vi "LDA_An_mx.vi"(0 "Board type":T1=enum."NI-DAQmx", 1 "interval scanning":bool, 2 "Client Time":dbl=3298049951.624875, 5 "No of samples+extra":i32=1024 min=0 step=1, 7 "Trigger mode":T2, 9 "output polarity":u16(ring)=1 items=["do not change", "positive", "negative"], 11 "Ch & spans":T3[](array[typedef]) {"low limit (-10V)" format="%.3f"; "high limit (10V)" format="%.3f"}, 12 "Actual Sampling rate (Hz)":dbl=100000.0 format="%.2f", 13 "Local Client?":bool=TRUE, 14 "Current Block No":i32) -> (3 "LDA Binary output":u16[][](array[numeric]), 4 "I16 Analogue data block":i16[][](array[numeric]), 6 "I16 TOF block (mu.s)":i16[](array[numeric]), 8 "Block Timings":T4={"Started"=3298049951.656125, "Ended"=3298049951.67175, "Analogue Frequency Hz"=100000.0} {"Analogue Frequency Hz" format="%.2f"}, 10 "group channel settings":T5(array[cluster]) {"scale offset" format="%#_16f"; "scale multiplier" format="%#_16f"; "input mode" format="%#_16f"; "coupling" format="%#_16f"; "gain" format="%#_16f"; "polarity" format="%#_16f"; "range" format="%#_16f"; "lower input limits" format="%#_16f"; "upper input limits" format="%#_16f"}, 15 "error out":errorcluster)   [LabVIEW 2011]
uses:
  PWAtasksGLOBAL.vi
  <vilib>/DAQmx/configure/timing.llb/DAQmx Timing (Sample Clock).vi
  <vilib>/DAQmx/create/channels.llb/DAQmx Create Channel (AI-Voltage-Basic).vi
  Globals/Meas_global.vi
  Controls/Block_start_and_end.ctl
  Applications/National Instruments/LabVIEW 2011/resource/objmgr/daqmx.rc
  <vilib>/DAQmx/read.llb/DAQmx Read (Analog 2D DBL NChan NSamp).vi
  Globals/LDA_meas_global_2.vi
  Controls/Ch_and_Spans.ctl
  Controls/Trigger_Mode.ctl
  Controls/Board_Types.ctl
panel:
  out "AI.Voltage.Rngs":dbl[](array[numeric])=[-10.0, 10.0]
  out "TotalSampPerChanAcquired":dbl=1024.0
  out "AvailSampPerChan":u32
  out "CurrReadPos":dbl=1024.0
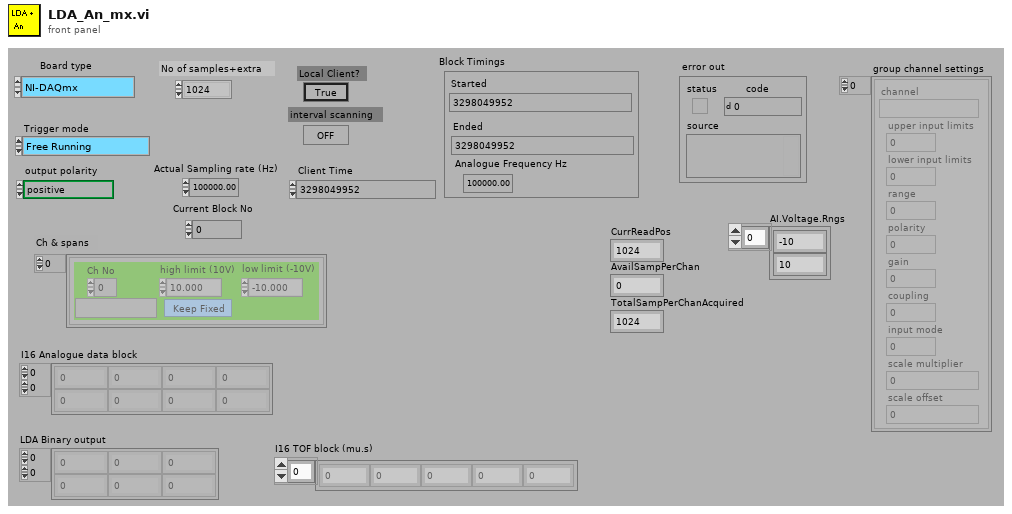
[diagram p1: front panel]
types:
  T1 = typedef "Board_Types.ctl" = enum16{"Simulate", "Local ADAM", "Server ADAM", "NI-DAQmx", "NI-DAQmxBase", "ADC488", "DT LV-link"}
  T2 = typedef "Trigger_Mode.ctl" = enum16{"Free Running", "Start on Trigger", "Trigger Every Block", "Trigger Every Sample"}
  T3 = typedef "Ch_and_Spans.ctl" = cluster{"high limit (10V)":sgl, "low limit (-10V)":sgl, "Ch No":i16, "Var name":string, "Use Latest Calib":bool}
  T4 = typedef "Block_start_and_end.ctl" = cluster{"Started":dbl, "Ended":dbl, "Analogue Frequency Hz":dbl}
  T5 = cluster{"channel":string, "upper input limits":sgl, "lower input limits":sgl, "range":sgl, "polarity":u16, "gain":sgl, "coupling":u16, "input mode":u16, "scale multiplier":dbl, "scale offset":dbl}[]
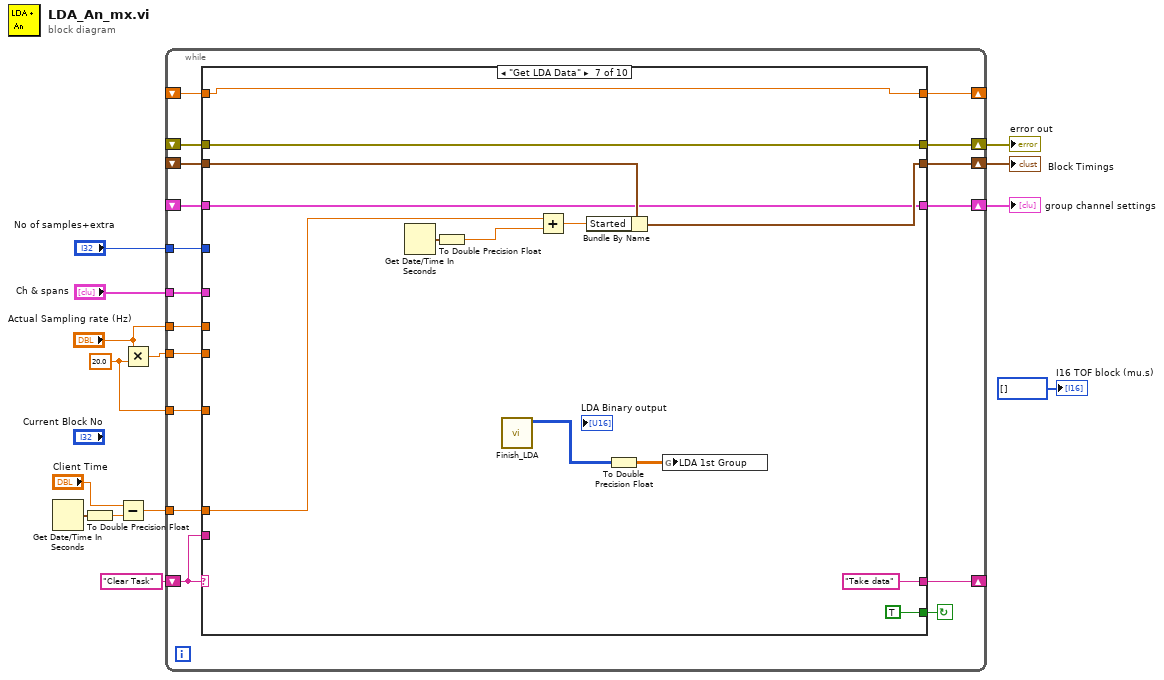
[diagram p0: block diagram]
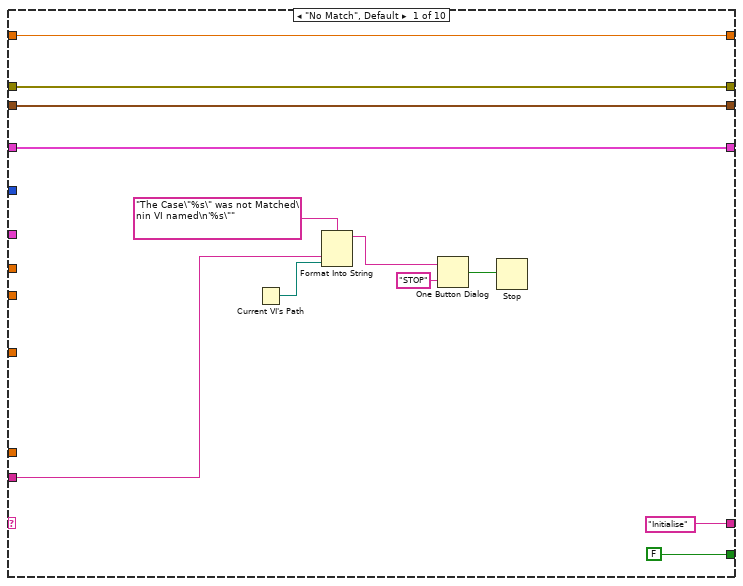
[diagram p2: hidden frame]
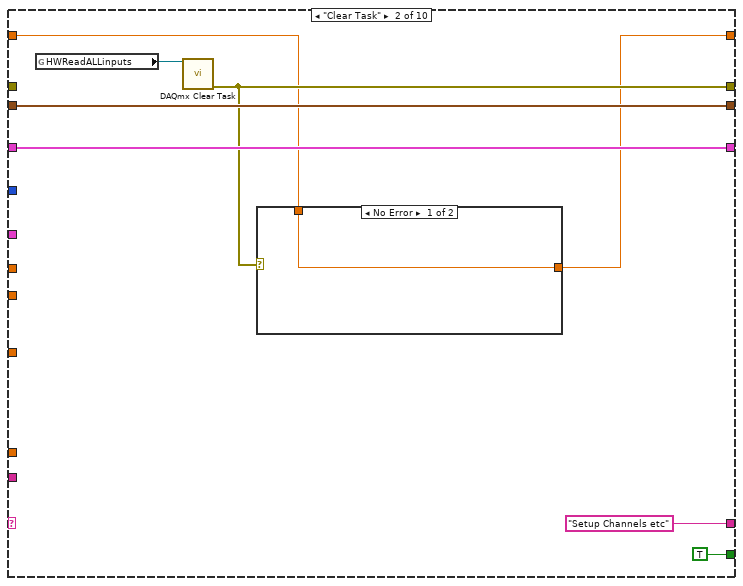
[diagram p3: hidden frame]
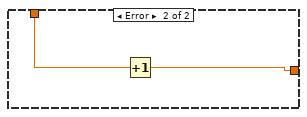
[diagram p4: hidden frame]
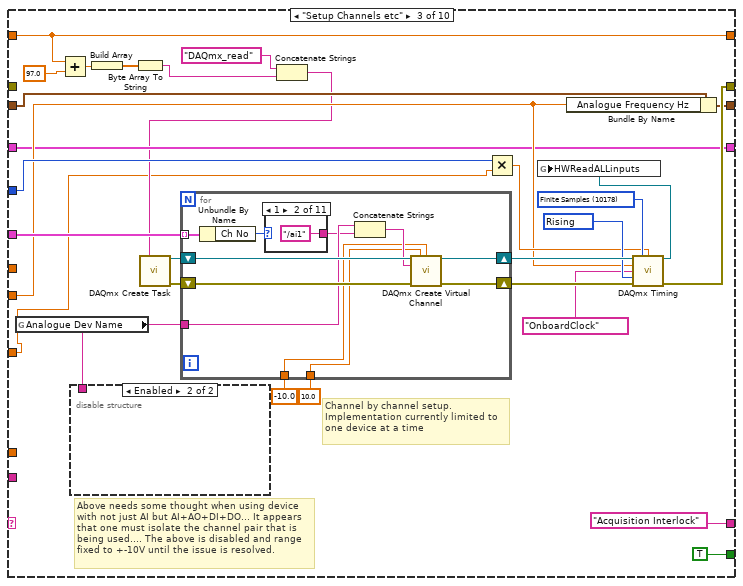
[diagram p5: hidden frame]
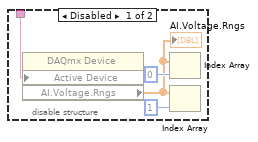
[diagram p6: hidden frame]
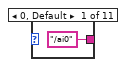
[diagram p7: hidden frame]
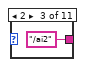
[diagram p8: hidden frame]
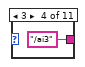
[diagram p9: hidden frame]
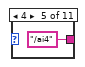
[diagram p10: hidden frame]
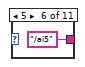
[diagram p11: hidden frame]
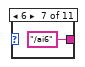
[diagram p12: hidden frame]
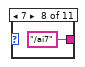
[diagram p13: hidden frame]
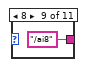
[diagram p14: hidden frame]
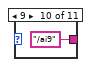
[diagram p15: hidden frame]
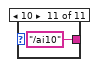
[diagram p16: hidden frame]
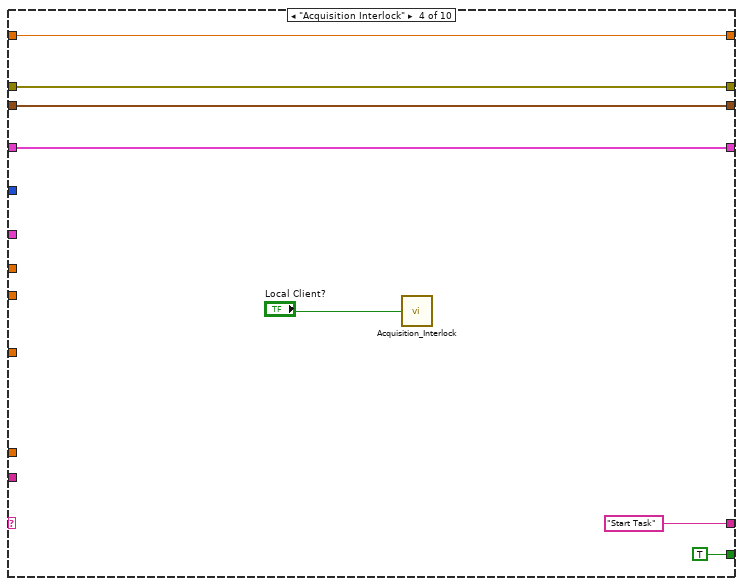
[diagram p17: hidden frame]
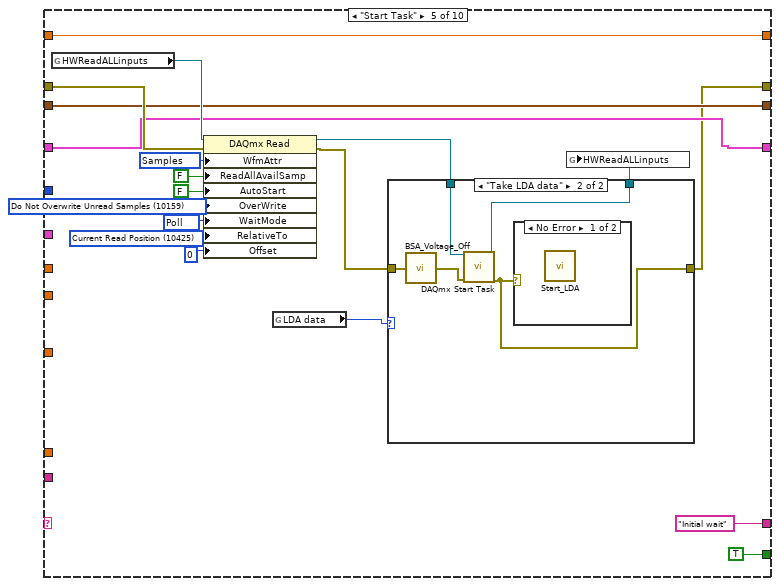
[diagram p18: hidden frame]
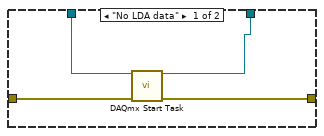
[diagram p19: hidden frame]
diagram:
  w1 = 20.0 ("y")
  n1 = Get Date/Time In Seconds() -> (seconds since 1Jan1904=w13:timestamp)
  n2 = To Double Precision Float(number=w13) -> (double precision float=w12:dbl)
  n3 = Subtract(x="Client Time", y=w12) -> (x-y=w10:dbl)
  n4 = Multiply(x="Actual Sampling rate (Hz)", y=w1) -> (x*y=w3:dbl)
  n5 = while {
    shift-left: "Clear Task" -> [w29]
    shift-right: [w30] -> _
    shift-right: [w21] -> w6
    shift-left: _ -> [w28]
    shift-right: [w20] -> w7
    shift-left: _ -> [w27]
    tunnel: w10 -> [w26]
    tunnel: w3 -> [w25]
    tunnel: "No of samples+extra" -> [w24]
    tunnel: "Ch & spans" -> [w23]
    shift-right: [w19] -> w5
    shift-left: _ -> [w22]
    shift-right: [w18] -> _
    shift-left: _ -> [w17]
    tunnel: "Actual Sampling rate (Hz)" -> [w16]
    tunnel: w1 -> [w15]
    stop <- w31 continue-if-true
    n6 = case shown="\"Get LDA Data\"" w29 {
      tunnel: [FALSE TRUE TRUE TRUE TRUE TRUE TRUE TRUE FALSE FALSE] -> w31
      tunnel: ["Initialise" "Setup Channels etc" "Acquisition Interlock" "Start Task" "Initial wait" "Get LDA Data" ("f") "Take data" "End Time" "End" ("f") "End" ("f")] -> w30
      tunnel: w29 -> [w38 _ _ _ _ _ _ _ _ _]
      tunnel: [w35 w46 w77 w114 w118 w153 w170 w190 w199 w212] -> w21
      tunnel: w28 -> [w35 _ _ w114 w126 w153 w170 w196 w199 w212]
      tunnel: [w33 w50 w75 w112 w125 w146 w174 w197 w205 T4 {"Started"=0.0, "Ended"=0.0, "Analogue Frequency Hz"=1000.0} ("Block Timings")] -> w20
      tunnel: w27 -> [w33 w50 w76 w112 w125 w147 w175 w197 w206 _]
      tunnel: w26 -> [_ _ _ _ _ w145 w172 _ w203 _]
      tunnel: w25 -> [_ _ w67 _ _ _ _ _ _ _]
      tunnel: w24 -> [_ _ w70 _ _ w159 _ w181 _ _]
      tunnel: w23 -> [_ _ w74 _ _ _ _ _ _ _]
      tunnel: [w34 w48 w66 w111 w123 w154 w168 w183 w200 w211] -> w19
      tunnel: w22 -> [w34 w48 w66 w111 w123 w154 w168 _ w200 w211]
      tunnel: [w32 w45 w56 w110 w122 w152 w166 w182 w198 w209] -> w18
      tunnel: w17 -> [w32 w44 w56 w110 w122 w152 w166 w182 w198 w209]
      tunnel: w16 -> [_ _ _ _ _ w151 _ _ _ _]
      tunnel: w15 -> [_ _ w55 _ _ _ _ w178 _ _]
      frame "No Match", Default {
        n7 = Current VI's Path() -> (path=w37:path)
        n8 = Format Into String(format string="The Case\"%s\" was not Matched\nin VI named\n'%s\"" ("Format String"), w38, w37) -> (resulting string=w41:string)  [unwired: 2 in, 1 out]
        n9 = One Button Dialog(message=w41, button name ("OK")="STOP") -> (true=w39:bool)
        n10 = Stop(stop? (T)=w39) -> ()
      }
      frame "Clear Task" {
        n11 = global read "PWAtasksGLOBAL.vi" "HWReadALLinputs"() -> (w47:refnum<k21>)
        n12 = call <vilib>:"DAQmx Clear Task.vi"("task in"=w47) -> ("error out"=w46:errorcluster)  [unwired: 1 in, 13 out]
        n13 = case shown="No Error" w46 {
          tunnel: [w52 w53] -> w45
          tunnel: w44 -> [w52 w54]
          frame No Error {
          }
          frame Error {
            n14 = Increment(x=w54) -> (x+1=w53:dbl)
          }
        }
      }
      frame "Setup Channels etc" {
        w72 = 10280 items=["Rising"=10280, "Falling"=10171] ("active edge")
        w80 = 10178 items=["Finite Samples"=10178, "Continuous Samples"=10123, "Hardware Timed Single Point"=12522] ("sample mode")
        # "Above needs some thought when using device with not just AI but AI+AO+DI+DO... It appears that one must isolate the channel pair that is being used.... The above is disabled and range fixed to +-10V until the issue is resolved."
        # "Channel by channel setup. Implementation currently limited to one device at a time"
        n15 = global read "PWAtasksGLOBAL.vi" "Analogue Dev Name"() -> (w63:string)
        n16 = Add(x=w56, y=97.0) -> (x+y=w61:dbl)
        n17 = disable-structure shown="Enabled" {
          disable-tunnel: w63 -> [w84 _]
          frame Disabled {
            n18 = property class="DAQmx Device"("Active Device"=w84) -> ("AI.Voltage.Rngs"=w85:dbl[])  [unwired: 2 in, 2 out]
            "AI.Voltage.Rngs" <- w85
            n19 = Index Array(array=w85, index=0) -> ()  [unwired: 1 out]
            n20 = Index Array(array=w85, index=1) -> ()  [unwired: 1 out]
          }
          frame Enabled {
          }
        }
        n21 = Build Array(w61) -> (w60:dbl[])
        n22 = Byte Array To String(unsigned byte array=w60) -> (string=w58:string)
        n23 = Concatenate Strings("DAQmx_read" ("new task name"), w58) -> (w57:string)
        n24 = call <vilib>:"DAQmx Create Task.vi"("new task name"=w57) -> ("task out"=w78:refnum<k21>, "error out"=w81:errorcluster)  [unwired: 4 in, 9 out]
        n25 = for {
          tunnel: w74 -> [w98] mode=indexing
          shift-right: [w96] -> w79
          shift-left: w78 -> [w97]
          shift-right: [w94] -> w82
          shift-left: w81 -> [w95]
          tunnel: w63 -> [w92]
          tunnel: -10.0 -> [w89]
          tunnel: 10.0 -> [w88]
          n26 = Unbundle By Name(w98) -> ("Ch No"=w93:i16)
          n27 = case shown="1" w93 {
            tunnel: ["/ai0" ("string") "/ai1" ("string") "/ai2" ("string") "/ai3" ("string") "/ai4" ("string") "/ai5" ("string") "/ai6" ("string") "/ai7" ("string") "/ai8" ("string") "/ai9" ("string") "/ai10" ("string")] -> w91
            frame 0, Default {
            }
            frame 1 {
            }
            frame 2 {
            }
            frame 3 {
            }
            frame 4 {
            }
            frame 5 {
            }
            frame 6 {
            }
            frame 7 {
            }
            frame 8 {
            }
            frame 9 {
            }
            frame 10 {
            }
          }
          n28 = Concatenate Strings(w92, w91) -> (w90:string)
          n29 = call-poly <vilib>:"DAQmx Create Virtual Channel.vi"("task in"=w97, "maximum value"=w88, "minimum value"=w89, "physical channels"=w90, "error in"=w95) -> ("task out"=w96:refnum<k21>, "error out"=w94:errorcluster)  [unwired: 4 in, 5 out]
        }
        n30 = Multiply(x=w70, y=w55) -> (x*y=w69:dbl)
        n31 = Bundle By Name(cluster=w76, "Analogue Frequency Hz"=w67) -> (w75:T4)
        n32 = call-poly <vilib>:"DAQmx Timing.vi"("task/channels in"=w79, "sample mode"=w80, "samples per channel"=w69, "rate"=w67, "source"=tag "OnboardClock", "active edge"=w72, "error in"=w82) -> ("task out"=w73:refnum<k21>, "error out"=w77:errorcluster)  [unwired: 7 out]
        n33 = global write "PWAtasksGLOBAL.vi" "HWReadALLinputs"(w73) -> ()
      }
      frame "Acquisition Interlock" {
        n34 = call "Acquisition_Interlock.vi"("Local Control"="Local Client?") -> ()
      }
      frame "Start Task" {
        w129 = 10425 items=["First Sample"=10424, "Current Read Position"=10425, "Reference Trigger"=10426, "First Pretrigger Sample"=10427, "Most Recent Sample"=10428] ("RelativeTo")
        w130 = 12524 items=["Wait For Interrupt"=12523, "Poll"=12524, "Yield"=12525, "Sleep"=12547] ("WaitMode")
        w131 = 10159 items=["Overwrite Unread Samples"=10252, "Do Not Overwrite Unread Samples"=10159] ("OverWrite")
        w133 = 10287 items=["Samples"=10287, "Samples and Timing"=10140, "Samples, Timing, and Attributes"=10141] ("WfmAttr")
        n35 = global read "PWAtasksGLOBAL.vi" "HWReadALLinputs"() -> (w127:refnum<k21>)
        n36 = property class="DAQmx Read"(reference=w127, error in=w126, "WfmAttr"=w133, "ReadAllAvailSamp"=FALSE, "AutoStart"=FALSE, "OverWrite"=w131, "WaitMode"=w130, "RelativeTo"=w129, "Offset"=0) -> (reference out=w119:refnum<k21>, error out=w120:errorcluster)
        n37 = global read "Meas_global.vi" "LDA data"() -> (w121:enum16{"No LDA data", "Take LDA data"})
        n38 = case shown="\"Take LDA data\"" w121 {
          tunnel: w120 -> [w139 w144]
          tunnel: [w136 w141] -> w118
          tunnel: w119 -> [w138 w142]
          tunnel: [w137 w140] -> w117
          frame "No LDA data" {
            n39 = call <vilib>:"DAQmx Start Task.vi"("task/channels in"=w138, "error in"=w139) -> ("task out"=w137:refnum<k21>, "error out"=w136:errorcluster)  [unwired: 12 out]
          }
          frame "Take LDA data" {
            n40 = call "BSA_Voltage_Off.vi"("error in"=w144) -> ("error out"=w143:errorcluster)
            n41 = call <vilib>:"DAQmx Start Task.vi"("task/channels in"=w142, "error in"=w143) -> ("task out"=w140:refnum<k21>, "error out"=w141:errorcluster)  [unwired: 12 out]
            n42 = case shown="No Error" w141 {
              frame No Error {
                n43 = call "Start_LDA.vi"() -> ()  [unwired: 1 out]
              }
              frame Error {
              }
            }
          }
        }
        n44 = global write "PWAtasksGLOBAL.vi" "HWReadALLinputs"(w117) -> ()
      }
      frame "Initial wait" {
        # "Wait for ONE block acquisition time. This is required when the calibration vi is running, probably due to an un-managed race condition"
        n45 = To Double Precision Float(number=w159) -> (double precision float=w160:dbl)
        n46 = Divide(x=w160, y=w151) -> (x/y=w158:dbl)
        n47 = Multiply(x=w158, y=1000.0) -> (x*y=w157:dbl)
        n48 = Round Toward +Infinity(x=w157) -> (ceil(x): smallest int >= x=w156:dbl)
        n49 = Get Date/Time In Seconds() -> (seconds since 1Jan1904=w150:timestamp)
        n50 = To Unsigned Long Integer(number=w156) -> (unsigned 32bit integer=w155:u32)
        n51 = To Double Precision Float(number=w150) -> (double precision float=w149:dbl)
        n52 = Wait (ms)(milliseconds to wait=w155) -> ()  [unwired: 1 out]
        n53 = Add(x=w145, y=w149) -> (x+y=w148:dbl)
        n54 = Bundle By Name(cluster=w147, "Started"=w148) -> (w146:T4)
      }
      frame "Get LDA Data" {
        n55 = Get Date/Time In Seconds() -> (seconds since 1Jan1904=w176:timestamp)
        n56 = To Double Precision Float(number=w176) -> (double precision float=w173:dbl)
        n57 = call "Finish_LDA.vi"() -> ("LDA Binary output"=w165:u16[][])  [unwired: 4 out]
        n58 = Add(x=w172, y=w173) -> (x+y=w171:dbl)
        n59 = Bundle By Name(cluster=w175, "Started"=w171) -> (w174:T4)
        n60 = To Double Precision Float(number=w165) -> (double precision float=w164:dbl[][])
        n61 = global write "LDA_meas_global_2.vi" "LDA 1st Group"(w164) -> ()
      }
      frame "Take data" {
        n62 = global read "PWAtasksGLOBAL.vi" "HWReadALLinputs"() -> (w188:refnum<k21>)
        n63 = Divide(x=w181, y=1.15) -> (x/y=w179:dbl)
        n64 = Multiply(x=w179, y=w178) -> (x*y=w177:dbl)
        n65 = call-poly <vilib>:"DAQmx Read.vi"("task/channels in"=w188, "number of samples per channel"=w177, "error in"=w196) -> ("task out"=w193:refnum<k21>, "data"=w185:dbl[][], "error out"=w187:errorcluster)  [unwired: 10 out]
        n66 = property class="DAQmx Read"(reference=w193, error in=w187) -> (reference out=w192:refnum<k21>, error out=w190:errorcluster, "CurrReadPos"=→"CurrReadPos":dbl, "AvailSampPerChan"=→"AvailSampPerChan":u32, "TotalSampPerChanAcquired"=→"TotalSampPerChanAcquired":dbl)
        n67 = global write "PWAtasksGLOBAL.vi" "HWReadALLinputs"(w192) -> ()
        n68 = call "Voltages_2_I16.vi"("Voltages"=w185) -> ("Group Channel Settings"=w183:T5, "I16 data"=→"I16 Analogue data block":i16[][])
      }
      frame "End Time" {
        # "Final transpose to get 2D data output correctly"
        n69 = Get Date/Time In Seconds() -> (seconds since 1Jan1904=w207:timestamp)
        n70 = To Double Precision Float(number=w207) -> (double precision float=w204:dbl)
        n71 = Add(x=w203, y=w204) -> (x+y=w202:dbl)
        n72 = Bundle By Name(cluster=w206, "Ended"=w202) -> (w205:T4)
      }
      frame "Extra case" {
      }
    }
  }
  "Block Timings" <- w7
  "error out" <- w6
  "group channel settings" <- w5
  "I16 TOF block (mu.s)" <- i16[] [] ("I16 TOF block (mu.s)")
